vi "Connection.vi"(4 "WriteTimeout [ms] (5000)":i32=5000, 6 "ReadTimeout [ms] (5000)":i32=5000, 7 "ReadMode (Standard)":T1(ring), 8 "error in (no error)":errorcluster, 9 "Port":u16, 10 "Address":string, 11 "Connection":refnum<k5>) -> (0 "error out":errorcluster, 3 "Connection":refnum<class "Connection.lvclass">)   [LabVIEW 2022 SP3, in "TcpSocket.lvlib" / "Connection.lvclass"]
uses:
  Connection.lvclass
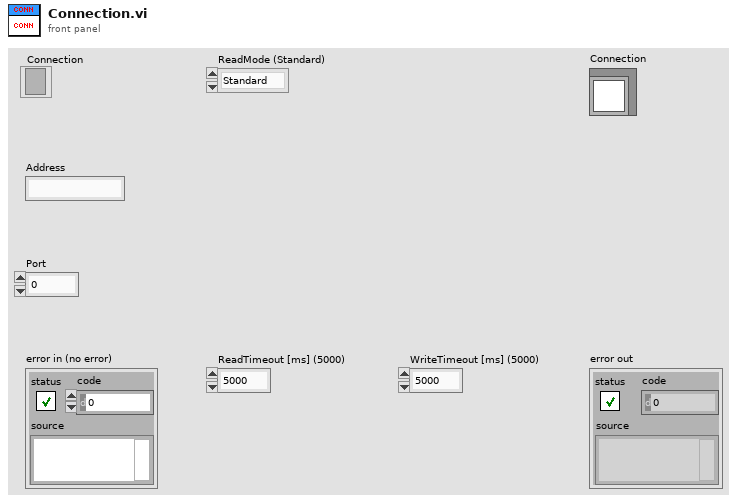
[diagram p1: front panel]
types:
  T1 = enum16{"Standard", "Buffered", "CRLF", "Immediate"}
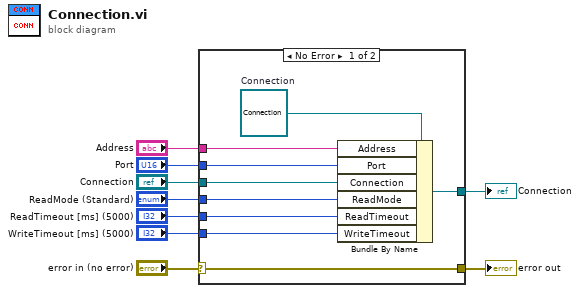
[diagram p0: block diagram]
diagram:
  n1 = case shown="No Error" "error in (no error)" {
    selector: "error in (no error)" -> [w18 w19]
    tunnel: [w18 w19] -> w8
    tunnel: [w17 _] -> w7
    tunnel: "Connection" -> [w16 _]
    tunnel: "Port" -> [w15 _]
    tunnel: "Address" -> [w14 _]
    tunnel: "ReadMode (Standard)" -> [w12 _]
    tunnel: "ReadTimeout [ms] (5000)" -> [w11 _]
    tunnel: "WriteTimeout [ms] (5000)" -> [w10 _]
    frame No Error {
      w13 = refnum<class "Connection.lvclass"> refnum  # Connection
      n2 = Bundle By Name(cluster=w13, "Address"=w14, "Port"=w15, "Connection"=w16, "ReadMode"=w12, "ReadTimeout"=w11, "WriteTimeout"=w10) -> (w17:refnum<class "Connection.lvclass">)
    }
    frame Error {
    }
  }
  "error out" <- w8
  "Connection" <- w7
